vi "New.vi"(8 "error in (no error)":errorcluster, 11 "Configuration":T1) -> (0 "error out":errorcluster, 3 "RandomNumberGenerator out":refnum<class "RandomNumberGenerator.lvclass">)   [LabVIEW 2020, in "RandomNumberGenerator.lvlib" / "RandomNumberGenerator.lvclass"]
doc: "<b>New</b>\nCreates a new instance of this plugin."
uses:
  RandomNumberGenerator.lvclass
  RandomNumberGenerator.lvclass/RandomNumberGenerator.ctl
  Configuration.ctl
panel:
  # "#via_ignore"
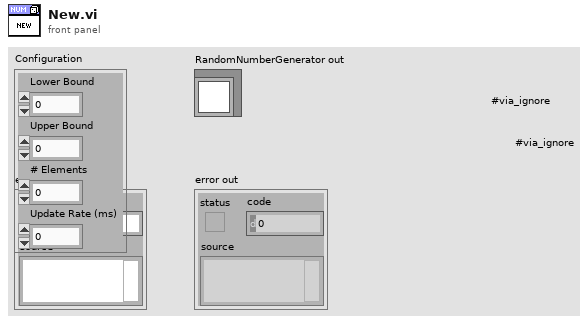
[diagram p1: front panel]
types:
  T1 = typedef "RandomNumberGenerator.lvlib/RandomNumberGenerator.lvclass/Configuration.ctl" = cluster{"Lower Bound":dbl, "Upper Bound":dbl, "# Elements":i32, "Update Rate (ms)":i32}
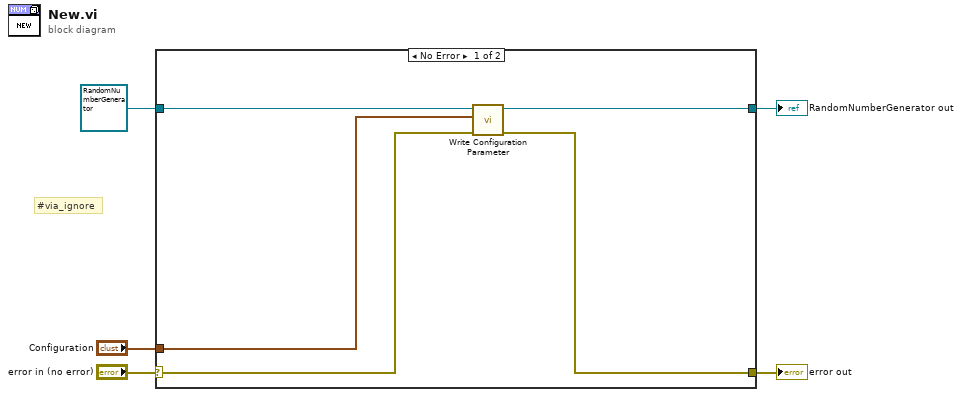
[diagram p0: block diagram]
diagram:
  # "#via_ignore"
  n1 = case shown="No Error" "error in (no error)" {
    selector: "error in (no error)" -> [w8 w12]
    tunnel: [w7 w12] -> w4
    tunnel: [w9 w11] -> w2
    tunnel: refnum<class "RandomNumberGenerator.lvclass"> refnum ("ADAS PE Template in") -> [w10 w11]
    tunnel: "Configuration" -> [w6 _]
    frame No Error {
      n2 = call "Write Configuration Parameter.vi"("error in (no error)"=w8, "Configuration"=w6, "RandomNumberGenerator in"=w10) -> ("error out"=w7:errorcluster, "RandomNumberGenerator out"=w9:refnum<class "RandomNumberGenerator.lvclass">)  [unwired: 7 in]
    }
    frame Error {
    }
  }
  "error out" <- w4
  "RandomNumberGenerator out" <- w2
